vi "euclidean distance.vi"(0 "X1":i8, 1 "X2":i8, 8 "error in (no error)":errorcluster) -> (9 "Result":i8, 10 "error out":errorcluster)   [LabVIEW 2011]
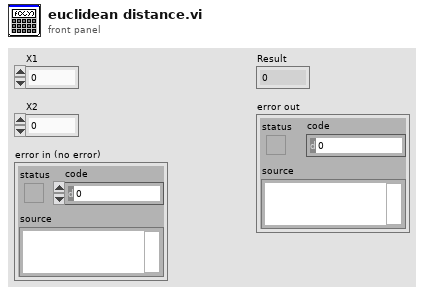
[diagram p1: front panel]
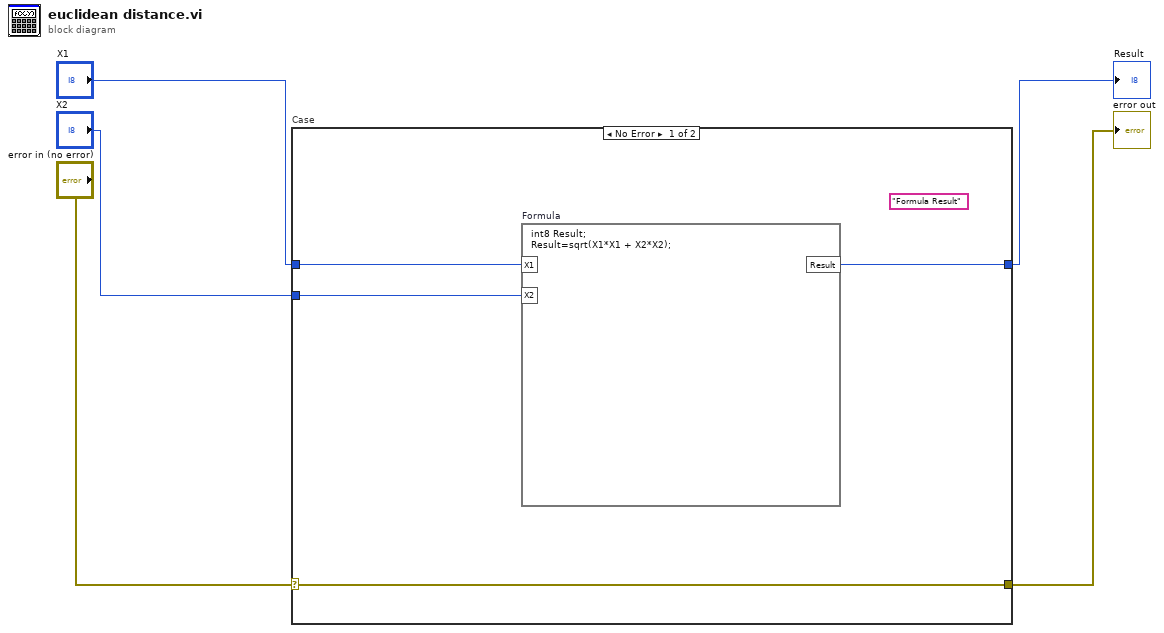
[diagram p0: block diagram]
diagram:
  n1 = case "Case" shown="No Error" "error in (no error)" {
    selector: "error in (no error)" -> [w6 w10]
    tunnel: [w7 _] -> w2
    tunnel: [w6 w10] -> w1
    tunnel: "X1" -> [w9 _]
    tunnel: "X2" -> [w8 _]
    frame No Error {
      (unwired) "Formula Result" ("Name Modifier")
      n2 = formula code="int8 Result;\nResult=sqrt(X1*X1 + X2*X2);"("X1"=w9, "X2"=w8) -> ("Result"=w7:i8)
    }
    frame Error {
    }
  }
  "Result" <- w2
  "error out" <- w1
